vi "Discover_MXG.vi"(8 "error in":errorcluster {"code" format="%.0x"}, 11 "Session In":refnum<visa-resource-name>="TCPIP0::10.0.1.24::inst0::INSTR") -> (0 "error out":errorcluster {"code" format="%.0x"}, 2 "Success?(t)":bool, 3 "Session Out":refnum<visa-resource-name>)   [LabVIEW 2018]
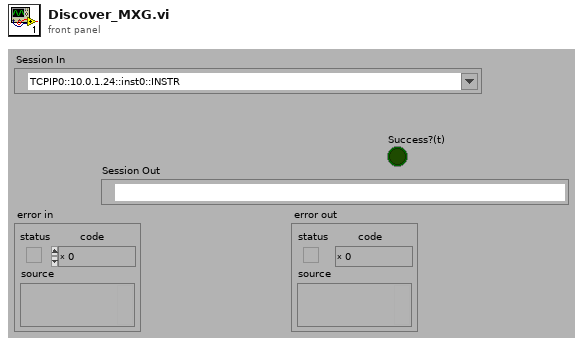
[diagram p1: front panel]
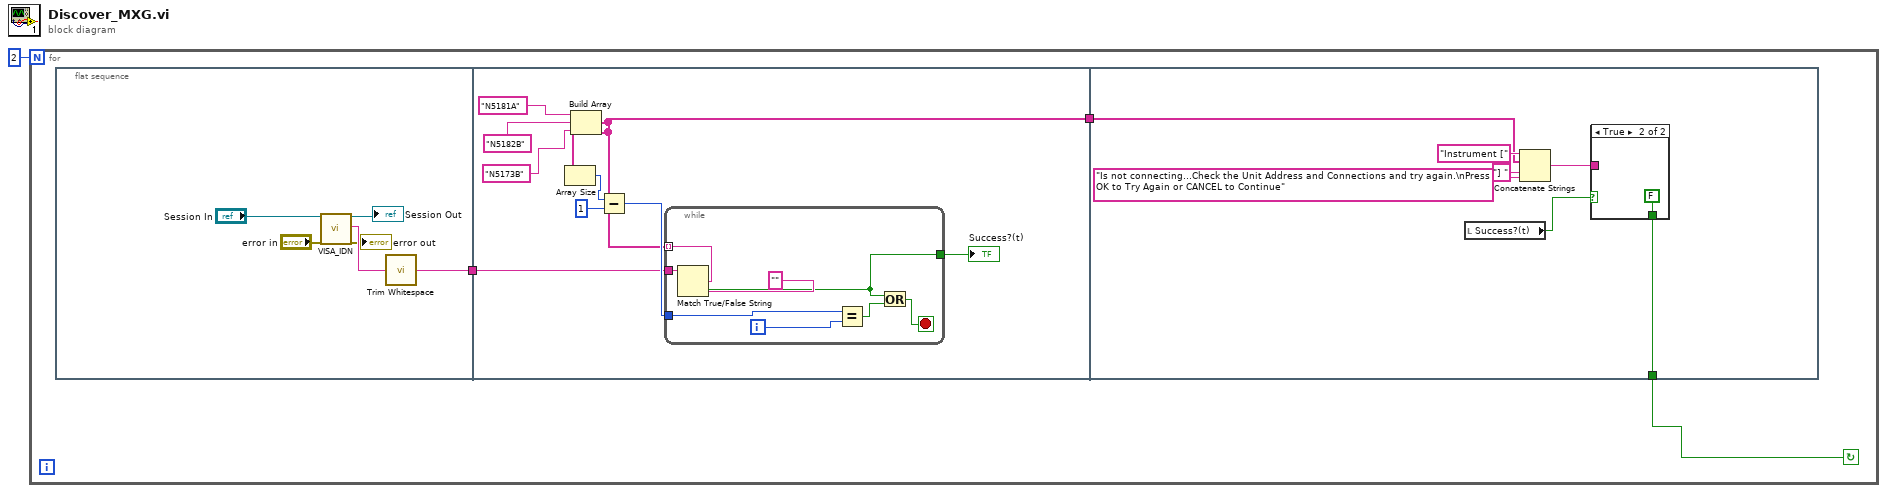
[diagram p0: block diagram]
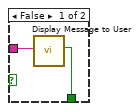
[diagram p2: hidden frame]
diagram:
  n1 = for {
    N: 2 -> [_]
    stop <- w2 continue-if-true
    n2 = flat-sequence {
      tunnel: [w7] -> w4
      tunnel: w4 -> [w15]
      tunnel: [w14] -> w3
      tunnel: w3 -> [w33]
      tunnel: [w28] -> w2
      frame #0 {
        n3 = call "VISA_IDN.vi"("Session In"="Session In", "error in"="error in") -> ("Session Out"=→"Session Out":refnum<visa-resource-name>, "Model"=w10:string, "error out"=→"error out":errorcluster)  [unwired: 11 in, 4 out]
        n4 = call <vilib>:"Trim Whitespace.vi"("string"=w10) -> ("trimmed string"=w7:string)  [unwired: 1 in]
      }
      frame #1 {
        n5 = Build Array("N5181A" ("element"), "N5182B" ("true string"), "N5173B" ("element")) -> (w14:string[])
        n6 = Array Size(array=w14) -> (size(s)=w18:i32)
        n7 = Subtract(x=w18, y=1) -> (x-y=w16:i32)
        n8 = while {
          tunnel: w14 -> [w26] mode=indexing
          tunnel: w15 -> [w25]
          tunnel: [w24] -> w19
          tunnel: w16 -> [w20]
          i -> [w21]
          stop <- w23 stop-if-true
          n9 = Match True/False String(2:"" ("false string"), 3:w26, 4:w25) -> (0:w24:bool)  [unwired: 1 out]
          n10 = Equal?(x=w20, y=w21) -> (x = y?=w22:bool)
          n11 = Or(x=w24, y=w22) -> (x .or. y?=w23:bool)
        }
        "Success?(t)" <- w19
      }
      frame #2 {
        n12 = local read "Success?(t)"() -> (w29:bool)
        n13 = Concatenate Strings("Instrument [" ("string"), w33, "] " ("string"), "Is not connecting...Check the Unit Address and Connections and try again.\nPress OK to Try Again or CANCEL to Continue" ("string")) -> (w30:string)
        n14 = case shown="True" w29 {
          tunnel: w30 -> [w36 _]
          tunnel: [w35 FALSE ("OK")] -> w28
          frame False {
            n15 = call "Display Message to User"("Message"=w36) -> ("OK"=w35:bool)  [unwired: 9 in, 1 out]
          }
          frame True {
          }
        }
      }
    }
  }
